vi "detector factors.vi"(7 "python in":refnum<k35>, 8 "error in":errorcluster, 9 "Line":T1, 10 "Line":dbl[][](array[numeric]), 11 "Source In":dbl[][](array[numeric])) -> (0 "error out":errorcluster, 3 "Line Factor":dbl[](array[numeric]), 5 "python out":refnum<k35>)   [LabVIEW 2023]
uses:
  control/sub_xraylib_lines.ctl
  python_to_labview/global python version.vi
panel:
  out "Array 2":dbl[](array[numeric])
  out "Array":i32[](array[numeric])
  out "XY Graph":cluster{"Source Out":dbl[], "Source Out":dbl[]}(graph)
  out "x*y 2":dbl
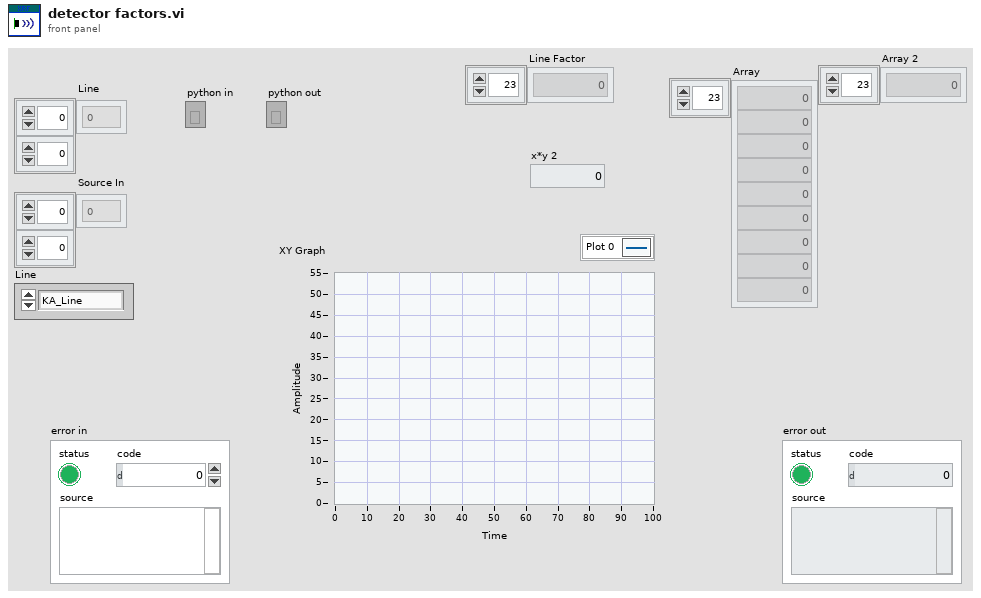
[diagram p1: front panel]
types:
  T1 = typedef "sub_xraylib_lines.ctl" = enum16{"KA_Line", "KB_Line", "LA_Line", "LB_Line", "KA1", "KA2", "KB1", "KB2", "KB3", "KB4", "KB5"}
  T2 = cluster{"detector-Kalpha":dbl[][], "detector-Kbeta":dbl[][], "detector-Lalpha":dbl[][]}
  T3 = cluster{"detector-Kalpha":dbl[], "detector-Kalpha":dbl[]}
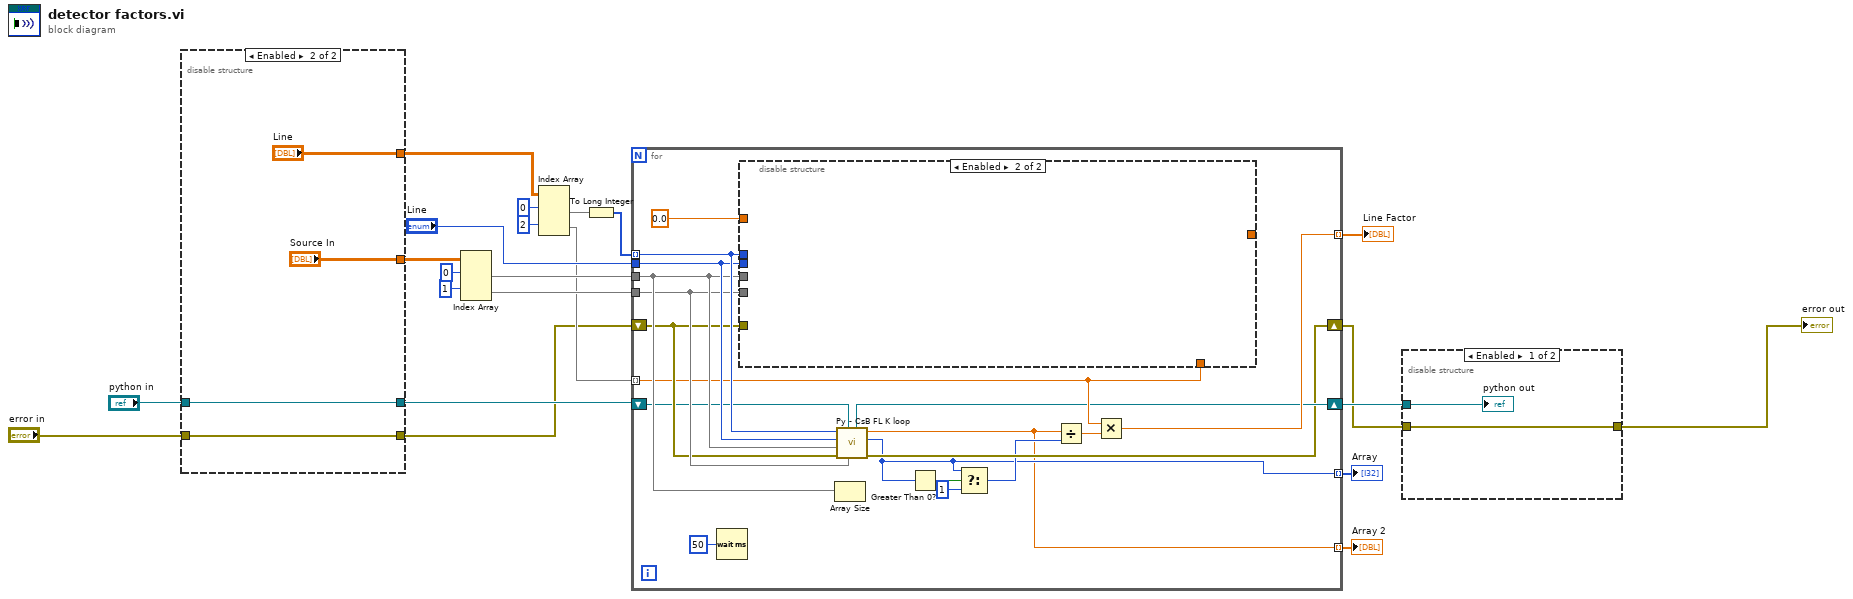
[diagram p0: block diagram]
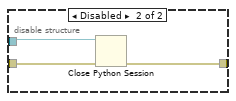
[diagram p2: hidden frame]
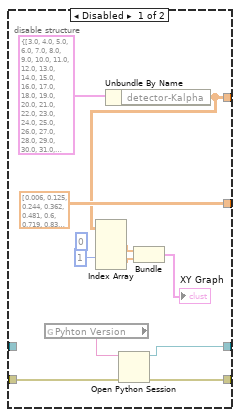
[diagram p3: hidden frame]
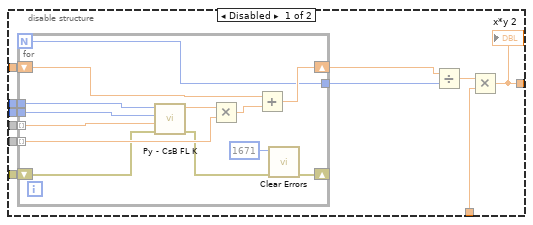
[diagram p4: hidden frame]
diagram:
  n1 = disable-structure shown="Enabled" {
    disable-tunnel: [w32 w37] -> w10
    disable-tunnel: "python in" -> [_ w37]
    disable-tunnel: "error in" -> [w31 w36]
    disable-tunnel: [w30 w36] -> w7
    disable-tunnel: [dbl[][] [[0.006, 0.125, 0.244, 0.362, 0.481, 0.6, 0.719, 0.838, 0.957, 1.075, 1.194, 1.313, 1.432, 1.551, 1.669, 1.788, 1.907, 2.026, 2.145, 2.263, 2.382, 2.501, 2.62, 2.739, 2.857, 2.976, 3.095, 3.214, 3.333, 3.451, 3.57, 3.689, 3.808, 3.927, 4.046, 4.164, 4.283, 4.402, 4.521, 4.64, 4.758, 4.877, 4.996, 5.115, 5.234, 5.352, 5.471, 5.59, 5.709, 5.828, 5.946, 6.065, 6.184, 6.303, 6.422, 6.54, 6.659, 6.778, 6.897, 7.016, 7.134, 7.253, 7.372, 7.491, 7.61, 7.729, 7.847, 7.966, 8.085, 8.204, 8.323, 8.441, 8.56, 8.679, 8.798, 8.917, 9.035, 9.154, 9.273, 9.392, 9.511, 9.629, 9.748, 9.867, 9.986, 10.105, 10.223, 10.342, 10.461, 10.58, 10.699, 10.818, 10.936, 11.055, 11.174, 11.293, 11.412, 11.53, 11.649, 11.768, 11.887, 12.006, 12.124, 12.243, 12.362, 12.481, 12.6, 12.718, 12.837, 12.956, 13.075, 13.194, 13.312, 13.431, 13.55, 13.669, 13.788, 13.906, 14.025, 14.144, 14.263, 14.382, 14.501, 14.619, 14.738, 14.857, 14.976, 15.095, 15.213, 15.332, 15.451, 15.57, 15.689, 15.807, 15.926, 16.045, 16.164, 16.283, 16.401, 16.52, 16.639, 16.758, 16.877, 16.995, 17.114, 17.233, 17.352, 17.471, 17.589, 17.708, 17.827, 17.946, 18.065, 18.184, 18.302, 18.421, 18.54, 18.659, 18.778, 18.896, 19.015, 19.134, 19.253, 19.372, 19.49, 19.609, 19.728, 19.847, 19.966, 20.084, 20.203, 20.322, 20.441, 20.56, 20.678, 20.797, 20.916, 21.035, 21.154, 21.273, 21.391, 21.51, 21.629, 21.748, 21.867, 21.985, 22.104, 22.223, 22.342, 22.461, 22.579, 22.698, 22.817, 22.936, 23.055, 23.173, 23.292, 23.411, 23.53, 23.649, 23.767, 23.886, 24.005, 24.124, 24.243, 24.361, 24.48, 24.599, 24.718, 24.837, 24.956, 25.074, 25.193, 25.312, 25.431, 25.55, 25.668, 25.787, 25.906, 26.025, 26.144, 26.262, 26.381, 26.5, 26.619, 26.738, 26.856, 26.975, 27.094, 27.213, 27.332, 27.45, 27.569, 27.688, 27.807, 27.926, 28.045, 28.163, 28.282, 28.401, 28.52, 28.639, 28.757, 28.876, 28.995, 29.114, 29.233, 29.351, 29.47, 29.589, 29.708, 29.827, 29.945, 30.064, 30.183, 30.302, 30.421, 30.539, 30.658, 30.777, 30.896, 31.015, 31.133, 31.252, 31.371, 31.49, 31.609, 31.728, 31.846, 31.965, 32.084, 32.203, 32.322, 32.44, 32.559, 32.678, 32.797, 32.916, 33.034, 33.153, 33.272, 33.391, 33.51, 33.628, 33.747, 33.866, 33.985, 34.104, 34.222, 34.341, 34.46, 34.579, 34.698, 34.817, 34.935, 35.054, 35.173, 35.292, 35.411, 35.529, 35.648, 35.767, 35.886, 36.005, 36.123, 36.242, 36.361, 36.48, 36.599, 36.717, 36.836, 36.955, 37.074, 37.193, 37.311, 37.43, 37.549, 37.668, 37.787, 37.905, 38.024, 38.143, 38.262, 38.381, 38.5, 38.618, 38.737, 38.856, 38.975, 39.094, 39.212, 39.331, 39.45, 39.569, 39.688, 39.806, 39.925, 40.044, 40.163, 40.282, 40.4, 40.519, 40.638, 40.757, 40.876, 40.994, 41.113, 41.232, 41.351, 41.47, 41.589, 41.707, 41.826, 41.945, 42.064, 42.183, 42.301, 42.42, 42.539, 42.658, 42.777, 42.895, 43.014, 43.133, 43.252, 43.371, 43.489, 43.608, 43.727, 43.846, 43.965, 44.083, 44.202, 44.321, 44.44, 44.559, 44.677, 44.796, 44.915, 45.034, 45.153, 45.272, 45.39, 45.509, 45.628, 45.747, 45.866, 45.984, 46.103, 46.222, 46.341, 46.46, 46.578, 46.697, 46.816, 46.935, 47.054, 47.172, 47.291, 47.41, 47.529, 47.648, 47.766, 47.885, 48.004], [0.0, 0.0, 0.0, 0.0, 0.0, 0.015886288, 0.017001115, 0.018115942, 0.013377926, 0.012820513, 0.009754738, 0.009754738, 0.008361204, 0.009476031, 0.004738016, 0.005574136, 0.004180602, 0.005574136, 0.003901895, 0.001672241, 0.002508361, 0.001393534, 0.001393534, 0.001672241, 0.00083612, 0.00083612, 0.00083612, 0.000557414, 0.000557414, 0.001114827, 0.000557414, 0.000557414, 0.001114827, 0.000557414, 0.0, 0.001114827, 0.000557414, 0.001393534, 0.001393534, 0.000557414, 0.001672241, 0.0, 0.0, 0.000557414, 0.000278707, 0.001114827, 0.00083612, 0.000557414, 0.00083612, 0.0, 0.000278707, 0.000557414, 0.00083612, 0.001672241, 0.001672241, 0.001114827, 0.000557414, 0.000557414, 0.000557414, 0.001672241, 0.0, 0.000557414, 0.000557414, 0.00083612, 0.000557414, 0.00083612, 0.001950948, 0.001672241, 0.00083612, 0.0, 0.000278707, 0.001672241, 0.001114827, 0.001114827, 0.001672241, 0.001950948, 0.003065775, 0.001672241, 0.001672241, 0.002787068, 0.003344482, 0.001672241, 0.003623188, 0.003065775, 0.006410256, 0.006410256, 0.003623188, 0.009197324, 0.009197324, 0.014492754, 0.011148272, 0.010869565, 0.017001115, 0.022017837, 0.019230769, 0.025083612, 0.026755853, 0.030936455, 0.032329989, 0.037625418, 0.039855072, 0.039855072, 0.046544036, 0.054347826, 0.060758082, 0.059643255, 0.066332219, 0.076365663, 0.073578595, 0.091415831, 0.090022297, 0.093088071, 0.095039019, 0.106187291, 0.102006689, 0.096432553, 0.13238573, 0.108138239, 0.122073579, 0.115105909, 0.127926421, 0.126532887, 0.118729097, 0.128762542, 0.140189521, 0.149386845, 0.143534002, 0.144648829, 0.139910814, 0.161371237, 0.151895206, 0.169175028, 0.16025641, 0.158026756, 0.157748049, 0.156354515, 0.164994426, 0.153010033, 0.160535117, 0.163322185, 0.172798216, 0.186733556, 0.334169454, 0.833890747, 1.0, 0.425027871, 0.177536232, 0.140189521, 0.160535117, 0.16722408, 0.139910814, 0.137123746, 0.14632107, 0.140746934, 0.14548495, 0.142976589, 0.135451505, 0.130434783, 0.133500557, 0.139910814, 0.223522854, 0.309643255, 0.211538462, 0.147714604, 0.127926421, 0.115384615, 0.095875139, 0.086956522, 0.083054627, 0.087513935, 0.076923077, 0.079431438, 0.085562988, 0.085841695, 0.066889632, 0.070791527, 0.073857302, 0.072742475, 0.061594203, 0.057692308, 0.059921962, 0.058528428, 0.04877369, 0.050724638, 0.044314381, 0.043478261, 0.04637709, 0.040477982, 0.032276477, 0.034284281, 0.03140524, 0.026690078, 0.023580546, 0.022762263, 0.0203534, 0.018996934, 0.017545987, 0.015505853, 0.013824136, 0.017546823, 0.014315496, 0.011837235, 0.011616778, 0.008314939, 0.009018395, 0.008144091, 0.008770067, 0.008326366, 0.007737737, 0.005871795, 0.004857302, 0.004470736, 0.003653846, 0.004576366, 0.003791249, 0.003676143, 0.003121516, 0.003085006, 0.002013099, 0.002437012, 0.0022932, 0.002105351, 0.001822464, 0.001806299, 0.002028986, 0.001497213, 0.001500279, 0.00155602, 0.00135786, 0.001133222, 0.00132107, 0.00110981, 0.000838071, 0.000931159, 0.001181438, 0.001139075, 0.001081661, 0.000890468, 0.001043757, 0.000795708, 0.000782609, 0.00099136, 0.000936176, 0.000991081, 0.000931717, 0.000980769, 0.000776198, 0.000841416, 0.000942586, 0.00095262, 0.000991639, 0.000792085, 0.00082748, 0.000816332, 0.000852564, 0.000895764, 0.000682553, 0.000951784, 0.000809922, 0.000903567, 0.00079738, 0.00084699, 0.000726867, 0.000759755, 0.001013099, 0.000869844, 0.00073913, 0.0008233, 0.000927536, 0.000784002, 0.000938127, 0.001008361, 0.000958194, 0.000843645, 0.000805463, 0.000759755, 0.000686455, 0.000858974, 0.00093757, 0.000828038, 0.000733556, 0.000785117, 0.000823857, 0.00089019, 0.000865663, 0.000744705, 0.0006767, 0.000754459, 0.000921962, 0.000805463, 0.000933389, 0.000797101, 0.00085786, 0.000740245, 0.000945931, 0.000983278, 0.000773133, 0.000853958, 0.000823579, 0.000761148, 0.000751394, 0.000782887, 0.000847826, 0.000916109, 0.000784002, 0.000762821, 0.001047659, 0.000965998, 0.000835006, 0.000828317, 0.000822185, 0.000906912, 0.000889075, 0.000723523, 0.000799331, 0.00078874, 0.000848105, 0.000845875, 0.000636566, 0.000705407, 0.000769509, 0.000738573, 0.00099136, 0.001016444, 0.00098913, 0.000871516, 0.000850613, 0.000698718, 0.000796265, 0.000857302, 0.000916945, 0.000739967, 0.000845318, 0.000609532, 0.000830825, 0.000901059, 0.001013935, 0.00102592, 0.000900223, 0.000837235, 0.000916667, 0.000911371, 0.000933946, 0.000747213, 0.000957079, 0.00091388, 0.000825808, 0.000919175, 0.000783166, 0.000781494, 0.000786789, 0.000759197, 0.000855909, 0.000769509, 0.000900223, 0.000815496, 0.000808528, 0.000786789, 0.000846433, 0.000951505, 0.000989409, 0.000830268, 0.000760591, 0.00082553, 0.000882107, 0.000989688, 0.000894091, 0.000771182, 0.000753623, 0.000761706, 0.000811873, 0.000836399, 0.000720178, 0.000809922, 0.000838907, 0.000879877, 0.000612319, 0.000960702, 0.000896042, 0.000713489, 0.000903846, 0.000924192, 0.000847547, 0.000890747, 0.000816332, 0.000905797, 0.000731327, 0.000911929, 0.000738016, 0.000902174, 0.000783724, 0.000673077, 0.000765329, 0.000922241, 0.000880435, 0.00058835, 0.00086204, 0.000822185, 0.000926143, 0.000930881, 0.000937848, 0.000952062, 0.000896042, 0.000981048, 0.000941193]] ("Source Out") "Source In"] -> w4
    disable-tunnel: [w23 "Line"] -> w3
    frame Disabled {
      (unwired) 0 ("index (row)")
      n2 = global read "global python version.vi" "Pyhton Version"() -> (w33:string)
      n3 = Unbundle By Name(T2 {"detector-Kalpha"=[[3.0, 4.0, 5.0, 6.0, 7.0, 8.0, 9.0, 10.0, 11.0, 12.0, 13.0, 14.0, 15.0, 16.0, 17.0, 18.0, 19.0, 20.0, 21.0, 22.0, 23.0, 24.0, 25.0, 26.0, 27.0, 28.0, 29.0, 30.0, 31.0, 32.0, 33.0, 34.0, 35.0, 36.0, 37.0, 38.0, 39.0, 40.0, 41.0, 42.0, 43.0, 44.0, 45.0, 46.0, 47.0, 48.0, 49.0, 50.0, 51.0, 52.0, 53.0, 54.0, 55.0, 56.0, 57.0, 58.0, 59.0, 60.0, 61.0, 62.0, 63.0, 64.0, 65.0, 66.0, 67.0, 68.0, 69.0, 70.0, 71.0, 72.0, 73.0, 74.0, 75.0, 76.0, 77.0, 78.0, 79.0, 80.0, 81.0, 82.0, 83.0, 84.0, 85.0, 86.0, 87.0, 88.0, 89.0, 90.0, 91.0, 92.0, 93.0, 94.0, 95.0], [0.0, 0.0, 0.0, 0.0, 0.3924, 0.5249, 0.6768, 0.8486, 1.04098, 1.2536, 1.4867, 1.73998, 2.0137, 2.30784, 2.62239, 2.9577, 3.3138, 3.69168, 4.0906, 4.51084, 4.9522, 5.41472, 5.89875, 6.40384, 6.93032, 7.47815, 8.04778, 8.63886, 9.25174, 9.88642, 10.54372, 11.2224, 11.9242, 12.649, 13.3953, 14.165, 14.9584, 15.7751, 16.6151, 17.47934, 18.3671, 19.2792, 20.2161, 21.1771, 22.16292, 23.1736, 24.2097, 25.2713, 26.3591, 27.4723, 28.612, 29.779, 30.9728, 32.1936, 33.4418, 34.7197, 36.0263, 37.361, 38.7247, 40.1181, 41.5422, 42.9962, 44.4816, 45.9984, 47.5467, 49.1277, 50.7416, 52.3889, 0.0, 0.0, 0.0, 0.0, 0.0, 0.0, 0.0, 0.0, 0.0, 0.0, 0.0, 0.0, 0.0, 0.0, 0.0, 0.0, 0.0, 0.0, 0.0, 0.0, 0.0, 0.0, 0.0, 0.0, 0.0], [0.0, 0.0, 0.0, 0.0, 0.2583308270676692, 0.3679172932330827, 0.4818499999999999, 0.5947372093023255, 0.6669925000000001, 0.7089211267605634, 0.7319703862660943, 0.7040022134387351, 0.7279737226277372, 0.7439912925170068, 0.7520104464285714, 0.7609919642857143, 0.7689955056179776, 0.7719974603174603, 0.7739979949874687, 0.774999619047619, 0.7760004319654428, 0.7769993952483801, 0.7779994834710744, 0.778, 0.779, 0.779, 0.779, 0.7780002368866329, 0.7730021207177814, 0.7619885106382979, 0.744007659574468, 0.7179823361823361, 0.6869892413793103, 0.648, 0.6079840259740259, 0.567, 0.5229794369645044, 0.48099535714285724, 0.44199583333333314, 0.4059869819819821, 0.37199671052631583, 0.3419944503735326, 0.31599739854318415, 0.29099787018255574, 0.27000170385395544, 0.24900830860534118, 0.2310052123552123, 0.21499751838235295, 0.20599919137466305, 0.1969976315789474, 0.188, 0.181, 0.17500100502512558, 0.16900196560196562, 0.16300096153846153, 0.15600164319248824, 0.14999842696629215, 0.143, 0.13600153958944283, 0.12899950842696634, 0.12199889958734525, 0.11399905787348588, 0.10700188425302824, 0.09899793415106518, 0.09100154938670107, 0.08300151802656547, 0.07500198265179676, 0.06700048573163327, 0.0, 0.0, 0.0, 0.0, 0.0, 0.0, 0.0, 0.0, 0.0, 0.0, 0.0, 0.0, 0.0, 0.0, 0.0, 0.0, 0.0, 0.0, 0.0, 0.0, 0.0, 0.0, 0.0, 0.0, 0.0]], "detector-Kbeta"=[[3.0, 4.0, 5.0, 6.0, 7.0, 8.0, 9.0, 10.0, 11.0, 12.0, 13.0, 14.0, 15.0, 16.0, 17.0, 18.0, 19.0, 20.0, 21.0, 22.0, 23.0, 24.0, 25.0, 26.0, 27.0, 28.0, 29.0, 30.0, 31.0, 32.0, 33.0, 34.0, 35.0, 36.0, 37.0, 38.0, 39.0, 40.0, 41.0, 42.0, 43.0, 44.0, 45.0, 46.0, 47.0, 48.0, 49.0, 50.0, 51.0, 52.0, 53.0, 54.0, 55.0, 56.0, 57.0, 58.0, 59.0, 60.0, 61.0, 62.0, 63.0, 64.0, 65.0, 66.0, 67.0, 68.0, 69.0, 70.0, 71.0, 72.0, 73.0, 74.0, 75.0, 76.0, 77.0, 78.0, 79.0, 80.0, 81.0, 82.0, 83.0, 84.0, 85.0, 86.0, 87.0, 88.0, 89.0, 90.0, 91.0, 92.0, 93.0, 94.0, 95.0], [0.0, 0.0, 0.0, 0.0, 0.0, 0.0, 0.0, 0.0, 1.0711, 1.3022, 1.55745, 1.83594, 2.1391, 2.46404, 2.8156, 3.1905, 3.5896, 4.0127, 4.4605, 4.93181, 5.42729, 5.94671, 6.49045, 7.05798, 7.64943, 8.26466, 8.90529, 9.572, 10.2642, 10.9821, 11.7262, 12.4959, 13.2914, 14.112, 14.9613, 15.8357, 16.7378, 17.6678, 18.6225, 19.6083, 20.619, 21.6568, 22.7236, 23.8187, 24.9424, 26.0955, 27.2759, 28.486, 29.7256, 30.9957, 32.2947, 33.624, 34.9869, 36.3782, 37.801, 39.2573, 40.7482, 42.2713, 43.826, 45.413, 47.0379, 48.697, 50.382, 52.119, 0.0, 0.0, 0.0, 0.0, 0.0, 0.0, 0.0, 0.0, 0.0, 0.0, 0.0, 0.0, 0.0, 0.0, 0.0, 0.0, 0.0, 0.0, 0.0, 0.0, 0.0, 0.0, 0.0, 0.0, 0.0, 0.0, 0.0, 0.0, 0.0], [0.0, 0.0, 0.0, 0.0, 0.0, 0.0, 0.0, 0.0, 0.6729352112676057, 0.713757939914163, 0.724203162055336, 0.712403503649635, 0.7348081632653061, 0.7479755414012739, 0.7571857142857142, 0.7662247191011237, 0.7711873015873016, 0.7736075187969925, 0.7748797619047619, 0.7759542176870748, 0.7770253925619834, 0.778, 0.7781643536121673, 0.779, 0.779, 0.7786334010152285, 0.7758279771615009, 0.7674479495268139, 0.751654103343465, 0.7271997050147492, 0.6957347578347578, 0.656235724137931, 0.6135549597855228, 0.5698220779220778, 0.5228303549571605, 0.4781817857142858, 0.43688333333333335, 0.3987711711711713, 0.36359539473684227, 0.3328625400213448, 0.305516129032258, 0.280781135902637, 0.25835548961424326, 0.23779864864864872, 0.21995532516493882, 0.2081796875, 0.1985857142857143, 0.18899473684210524, 0.18132030848329048, 0.17488845208845208, 0.1685158653846154, 0.16200312989045385, 0.1547738131699847, 0.1481532584269663, 0.14074193548387093, 0.13332512562814075, 0.12590210674157304, 0.11798734525447048, 0.11009017496635262, 0.10208707124010556, 0.09362930923176242, 0.0851808981657179, 0.07678438661710038, 0.06831147540983608, 0.0, 0.0, 0.0, 0.0, 0.0, 0.0, 0.0, 0.0, 0.0, 0.0, 0.0, 0.0, 0.0, 0.0, 0.0, 0.0, 0.0, 0.0, 0.0, 0.0, 0.0, 0.0, 0.0, 0.0, 0.0, 0.0, 0.0, 0.0, 0.0]], "detector-Lalpha"=[[3.0, 4.0, 5.0, 6.0, 7.0, 8.0, 9.0, 10.0, 11.0, 12.0, 13.0, 14.0, 15.0, 16.0, 17.0, 18.0, 19.0, 20.0, 21.0, 22.0, 23.0, 24.0, 25.0, 26.0, 27.0, 28.0, 29.0, 30.0, 31.0, 32.0, 33.0, 34.0, 35.0, 36.0, 37.0, 38.0, 39.0, 40.0, 41.0, 42.0, 43.0, 44.0, 45.0, 46.0, 47.0, 48.0, 49.0, 50.0, 51.0, 52.0, 53.0, 54.0, 55.0, 56.0, 57.0, 58.0, 59.0, 60.0, 61.0, 62.0, 63.0, 64.0, 65.0, 66.0, 67.0, 68.0, 69.0, 70.0, 71.0, 72.0, 73.0, 74.0, 75.0, 76.0, 77.0, 78.0, 79.0, 80.0, 81.0, 82.0, 83.0, 84.0, 85.0, 86.0, 87.0, 88.0, 89.0, 90.0, 91.0, 92.0, 93.0, 94.0, 95.0], [0.0, 0.0, 0.0, 0.0, 0.0, 0.0, 0.0, 0.0, 0.0, 0.0, 0.0, 0.0, 0.0, 0.0, 0.0, 0.0, 0.0, 0.0, 0.3954, 0.4522, 0.5113, 0.5728, 0.6374, 0.705, 0.7762, 0.8515, 0.9297, 1.0117, 1.09792, 1.188, 1.282, 1.3791, 1.48043, 1.586, 1.69413, 1.80656, 1.92256, 2.04236, 2.16589, 2.29316, 2.424, 2.55855, 2.69674, 2.83861, 2.98431, 3.13373, 3.28694, 3.44398, 3.60472, 3.76933, 3.93765, 4.1099, 4.2865, 4.46626, 4.65097, 4.8402, 5.0337, 5.2304, 5.4325, 5.6361, 5.8457, 6.0572, 6.2728, 6.4952, 6.7198, 6.9487, 7.1799, 7.4156, 7.6555, 7.899, 8.1461, 8.3976, 8.6525, 8.9117, 9.1751, 9.4423, 9.7133, 9.9888, 10.2685, 10.5515, 10.8388, 11.1308, 11.4268, 11.727, 12.0313, 12.3397, 12.652, 12.9687, 13.2907, 13.6147, 13.9441, 14.2786, 14.6172], [0.0, 0.0, 0.0, 0.0, 0.0, 0.0, 0.0, 0.0, 0.0, 0.0, 0.0, 0.0, 0.0, 0.0, 0.0, 0.0, 0.0, 0.0, 0.26081203007518794, 0.3077894736842105, 0.3566691729323308, 0.40384999999999993, 0.4522999999999999, 0.5003953488372093, 0.5471720930232558, 0.5959375, 0.6252625, 0.6560125000000001, 0.678223661971831, 0.6959859154929577, 0.7117639484978541, 0.7213489270386266, 0.7313514592274678, 0.7210434782608696, 0.7090765217391304, 0.7098300729927007, 0.7199906569343065, 0.7295434013605442, 0.7362661224489796, 0.7431923809523809, 0.7469554140127389, 0.7503834394904458, 0.7540019642857143, 0.7578020535714286, 0.7615912359550562, 0.7649489887640449, 0.7683919101123595, 0.7700315873015873, 0.7713073015873017, 0.7723876190476191, 0.773231328320802, 0.774045, 0.7744654761904762, 0.7748934761904762, 0.7753173922902494, 0.775746485260771, 0.7761764578833693, 0.7766012958963283, 0.7770361570247935, 0.7774568181818182, 0.7778898760330579, 0.778, 0.778, 0.7781733840304182, 0.7786003802281369, 0.779, 0.779, 0.779, 0.779, 0.779, 0.7788340101522843, 0.7784084602368867, 0.7778898858075041, 0.7757756933115824, 0.7736272430668842, 0.7696982649842272, 0.7649963722397476, 0.7591878419452888, 0.7515364741641337, 0.743712389380531, 0.7326949852507374, 0.7214973451327433, 0.7089561253561254, 0.6956994301994301, 0.6812280000000001, 0.6646382068965516, 0.6478391420911529, 0.630857908847185, 0.6135924932975871, 0.5963016883116884, 0.5787622077922077, 0.56069684741488, 0.5419094577553594]]} ("detector-lines")) -> ("detector-Kalpha"=w23:dbl[][])
      n4 = Index Array(array=w23, index (row) #2=1 ("index (row)")) -> (element #1=w26:dbl[], element #2=w25:dbl[])  [unwired: 3 in]
      n5 = Open Python Session(python version=w33, 3:w31) -> (session out=w32:refnum<k35>, error out=w30:errorcluster)  [unwired: 1 in]
      n6 = Bundle("detector-Kalpha"=w26, "detector-Kalpha"=w25) -> (→"XY Graph":T3)  [unwired: 1 in]
    }
    frame Enabled {
    }
  }
  n7 = Index Array(array=w4, index (row) #1=0 ("index (row)"), index (row) #2=1 ("index (row)")) -> (element #1=w21:dbl[], element #2=w19:dbl[])  [unwired: 2 in]
  n8 = Index Array(array=w3, index (row) #1=0 ("index (row)"), index (row) #2=2 ("index (row)")) -> (element #1=w15:dbl[], element #2=w13:dbl[])  [unwired: 2 in]
  n9 = To Long Integer(number=w15) -> (32bit integer=w14:i32[])
  n10 = for {
    tunnel: w21 -> [w52]
    tunnel: w19 -> [w51]
    tunnel: "Line" -> [w53]
    tunnel: w14 -> [w54] mode=indexing
    tunnel: w13 -> [w48] mode=indexing
    tunnel: [w47] -> w12 mode=indexing
    shift-right: [w43] -> w6
    shift-left: w7 -> [w50]
    shift-right: [w45] -> w11
    shift-left: w10 -> [w46]
    tunnel: [w39] -> w2 mode=indexing
    tunnel: [w38] -> w1 mode=indexing
    n11 = Wait (ms)(milliseconds to wait=u32 50) -> ()  [unwired: 1 out]
    n12 = disable-structure shown="Enabled" {
      disable-tunnel: 0.0 -> [w66 _]
      disable-tunnel: [w62 _] -> _
      disable-tunnel: w54 -> [w61 _]
      disable-tunnel: w53 -> [w60 _]
      disable-tunnel: w52 -> [w59 _]
      disable-tunnel: w51 -> [w58 _]
      disable-tunnel: w50 -> [w57 _]
      disable-tunnel: w48 -> [w56 _]
      frame Disabled {
        n13 = for {
          N -> [w75]
          tunnel: w59 -> [w71] mode=indexing
          tunnel: w58 -> [w79] mode=indexing
          shift-right: [w77] -> w64
          shift-left: w66 -> [w76]
          tunnel: w60 -> [w70]
          tunnel: w61 -> [w69]
          tunnel: [w75] -> w65
          shift-right: [w74] -> _
          shift-left: w57 -> [w72]
          n14 = call "Py - CsB FL K.vi"("error in"=w72, "En"=w71, "Lin"=w70, "Z"=w69) -> ("error out"=w68:errorcluster, "CsB FL K"=w67:dbl)  [unwired: 6 in]
          n15 = Multiply(x=w67, y=w79) -> (x*y=w78:dbl)
          n16 = Add(x=w76, y=w78) -> (x+y=w77:dbl)
          n17 = call <vilib>:"Clear Errors.vi"("error in (no error)"=w68, "specific error code to clear (0: all)"=1671) -> ("error out"=w74:errorcluster)  [unwired: 4 in, 1 out]
        }
        n18 = Divide(x=w64, y=w65) -> (x/y=w63:dbl)
        n19 = Multiply(x=w63, y=w56) -> (x*y=w62:dbl)
        "x*y 2" <- w62
      }
      frame Enabled {
      }
    }
    n20 = Array Size(array=w52) -> ()  [unwired: 1 out]
    n21 = call "Py - CsB FL K loop.vi"("Int_array"=w51, "python in"=w46, "error in"=w50, "En_array"=w52, "Lin"=w53, "Z"=w54) -> ("error out"=w43:errorcluster, "Num Iterations"=w39:i32, "CsB FL K"=w38:dbl, "python out"=w45:refnum<k35>)  [unwired: 2 in]
    n22 = Greater Than 0?(x=w39) -> (x > 0?=w42:bool)
    n23 = Select(t=w39, s=w42, f=1) -> (s? t:f=w41:i32)
    n24 = Divide(x=w38, y=w41) -> (x/y=w49:dbl)
    n25 = Multiply(x=w48, y=w49) -> (x*y=w47:dbl)
  }
  "Line Factor" <- w12
  "Array" <- w2
  "Array 2" <- w1
  n26 = disable-structure shown="Enabled" {
    disable-tunnel: w11 -> [w81 w84]
    disable-tunnel: w6 -> [w80 w83]
    disable-tunnel: [w80 w82] -> w5
    frame Enabled {
      "python out" <- w81
    }
    frame Disabled {
      n27 = Close Python Session(session in=w84, error in=w83) -> (11:w82:errorcluster)
    }
  }
  "error out" <- w5
